vi "PXIe-SG.vi"() -> (0 "error out":errorcluster)   [LabVIEW 2022 SP3]
uses:
  Device ID port info.ctl
  Sub_vis/Upload Data.ctl
  <vilib>/DAQmx/read.llb/DAQmx Read (Analog 2D DBL NChan NSamp).vi
  Globals/Meas_global.vi
  <vilib>/DAQmx/miscellaneous.llb/DAQmx Fill In Error Info.vi
  <resource>/objmgr/daqmx.rc
panel:
  out "combinedTasks":string[](array[string])
  out "Device port info":T1[](array[typedef])
  out "FsReq":dbl=2000.0
  out "FsRead":dbl=2000.0000006348273 format="%#_11g"
  out "AuditTrail":string[](array[string])=["Clear Task", "Setup Channels etc", "Start Task", "Take data", "End"]
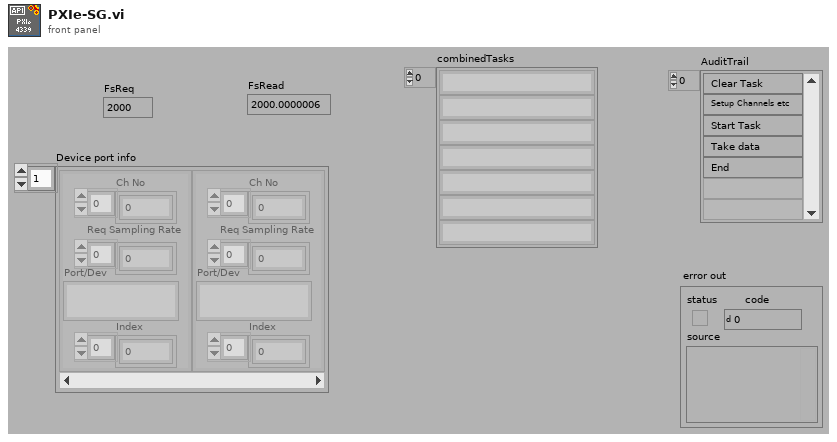
[diagram p1: front panel]
types:
  T1 = typedef "Device ID port info.ctl" = cluster{"Ch No":i16[], "Req Sampling Rate":dbl[], "Port":string, "Index":i32[]}
  T2 = typedef "Analysis_info_cluster.ctl" = cluster{"Colour":u32, "Inst type":T3, "Inst name":string, "Symbol":string, "Code name":string, "Extra Info":string, "Inst Array":T4, "U":dbl, "u^2":dbl, "u^3":dbl, "u^4":dbl, "Skew_u":dbl, "Kurt_u":dbl, "Sd Error in Mean":dbl, "% u'/U":dbl, "X":dbl, "Y":dbl, "Z":dbl, "Timescale integral Estimate":dbl, "Sd Error in Variance":dbl, "Calib File":path, "Calib Constants":dbl[], "Output Position":bool, "Stats":enum16{"None", "Basic", "Full"}, "Av Sampling Rate":dbl, "Av No of Samples":dbl, "Total Meas Time (s)":dbl, "OrigChName":string, "Max value":dbl, "Min value":dbl, "Req Sample Rate Hz":dbl, "Sync Delay Time (s)":dbl, "Ch No":i16, "Device":string, "Use Latest Calib":bool, "Port":string, "Metadata Ch Names":string[], "Metadata Ch Values":string[], "Label":string, "chState":T5, "Point Drift":dbl, "inputConfig":string}
  T3 = typedef "Inst_type.ctl" = enum16{"Raw voltage", "Raw with zero offsetting", "Propeller anemometer", "Pressure Transducer", "Pitot-static tube", "Hot wire", "Cross wire 1", "Cross wire 2", "Generic Linear", "Generic Polynomial", "Generic BackPoly", "Fast FID", "Thermocouple", "Cold wire", "Pulsed Wire", "LDA Vel", "LDA Tran time", "LDA Arr time", "Microphone"}
  T4 = typedef "Instrument_Array.ctl" = enum16{"PWA", "LDA", "Analogue"}
  T5 = typedef "channelState.ctl" = enum32{"No Selection", "Solo", "Mute"}
  T6 = typedef "Upload Data.ctl" = enum16{"Voltage Array", "Time Trace Cluster"}
  T7 = typedef "Rendezvous RefNum" = refnum<k1>
  T8 = typedef "Setup.ctl" = enum16{"Run Program", "Show Setup", "Save Current Setup", "Setup Front Panel"}
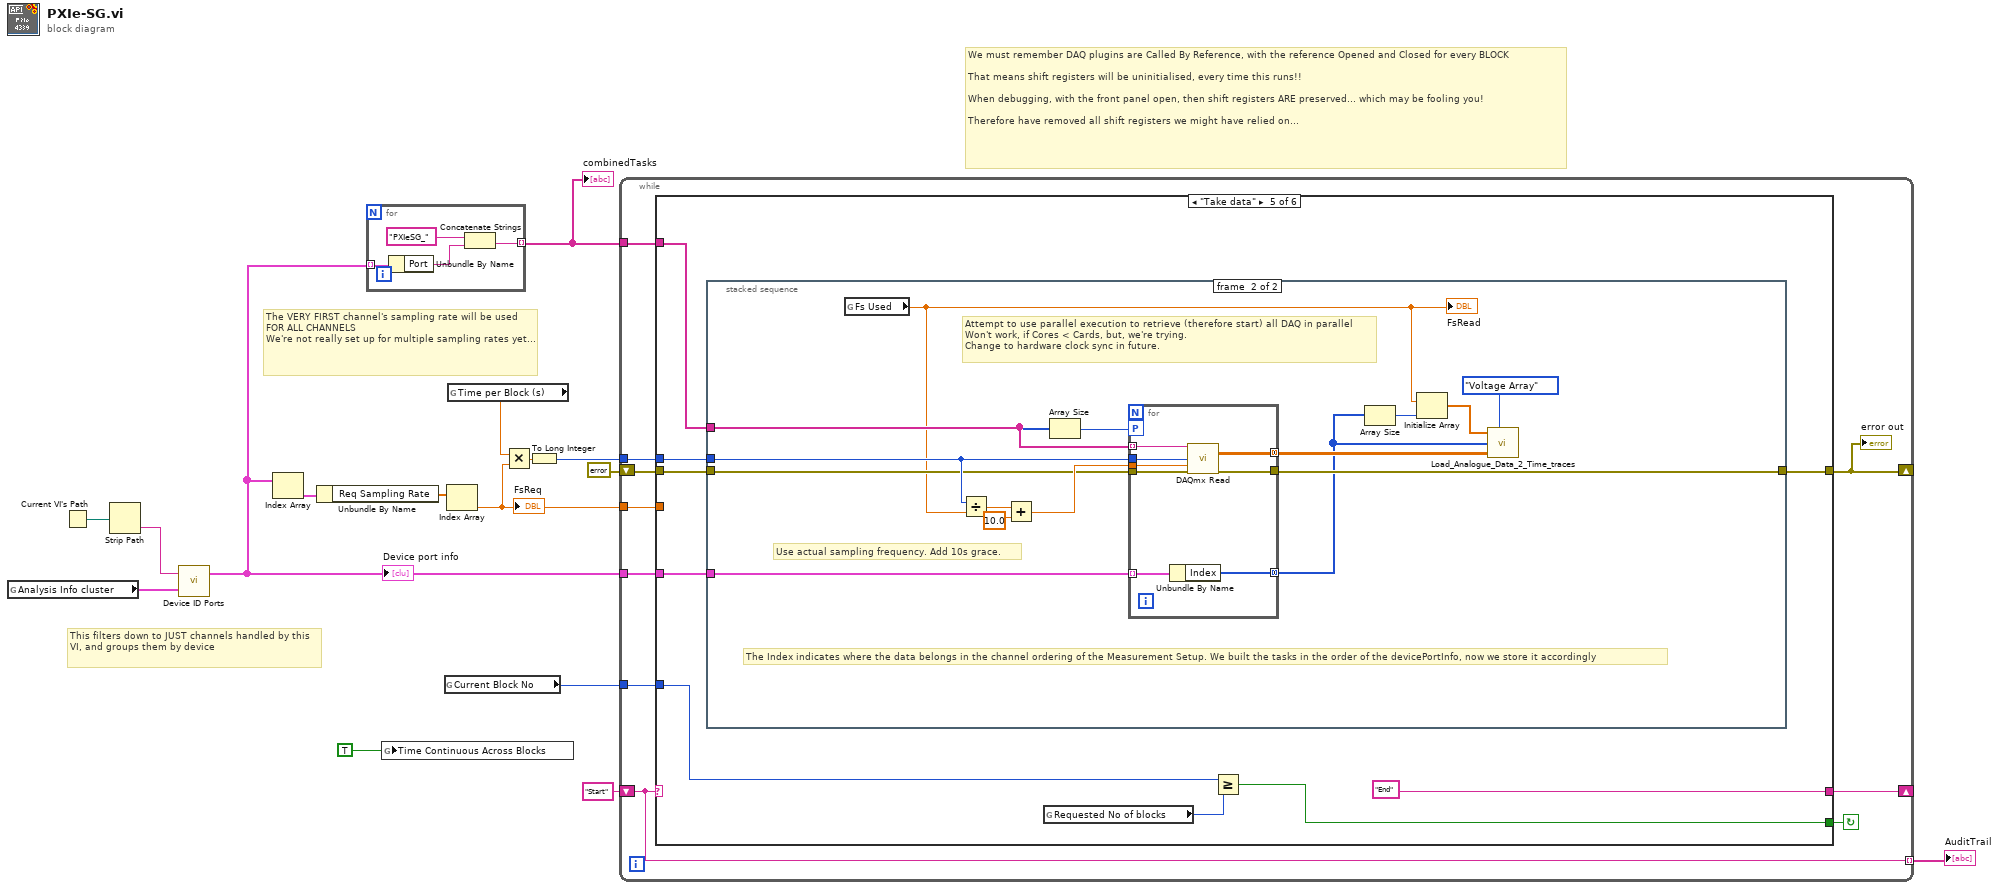
[diagram p0: block diagram]
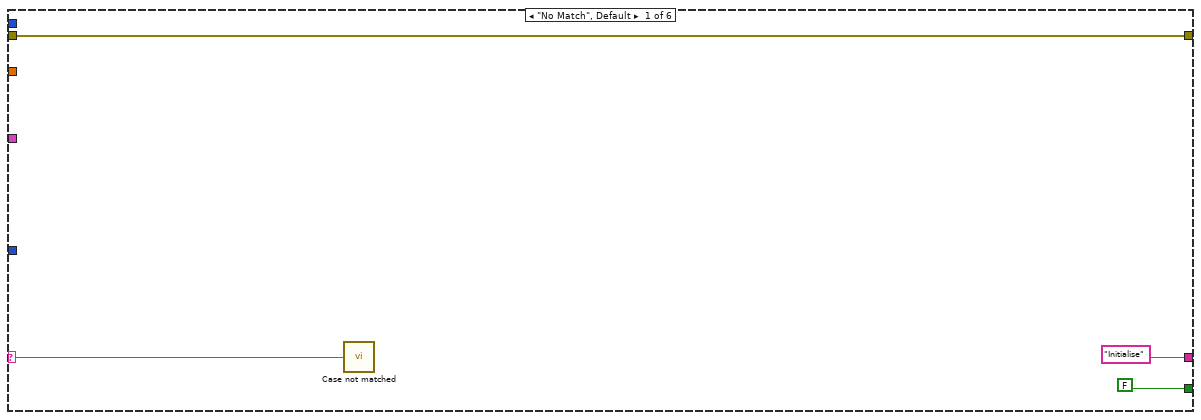
[diagram p2: hidden frame]
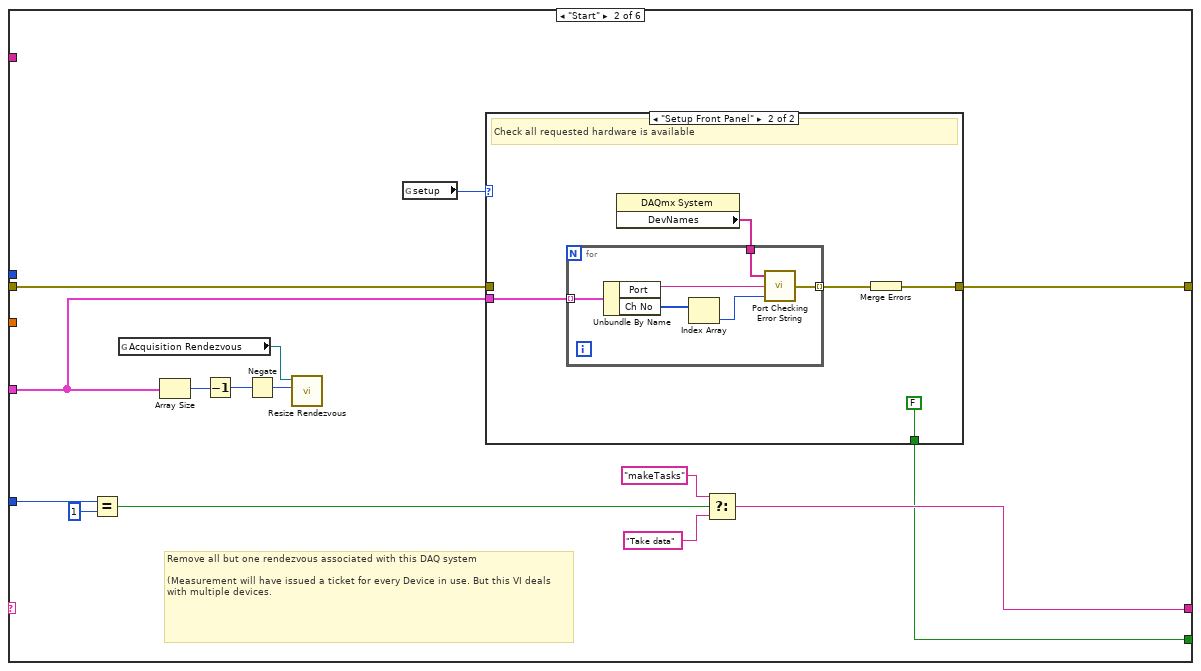
[diagram p3: hidden frame]
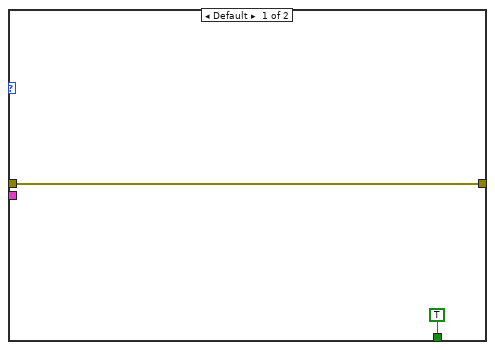
[diagram p4: hidden frame]
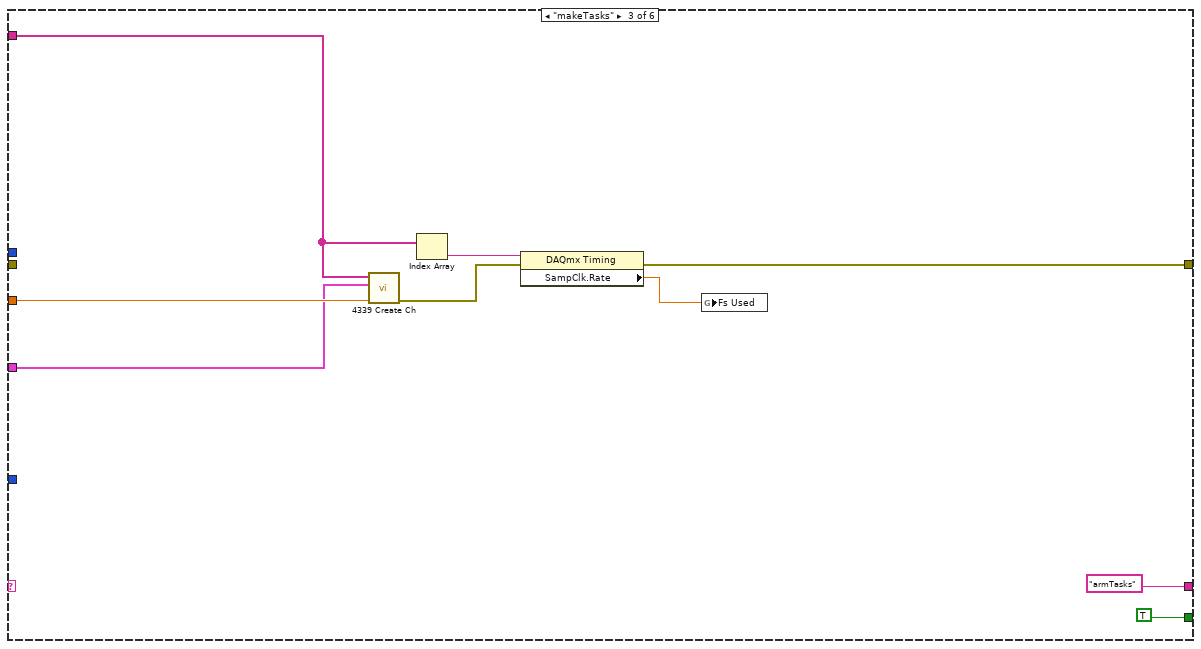
[diagram p5: hidden frame]
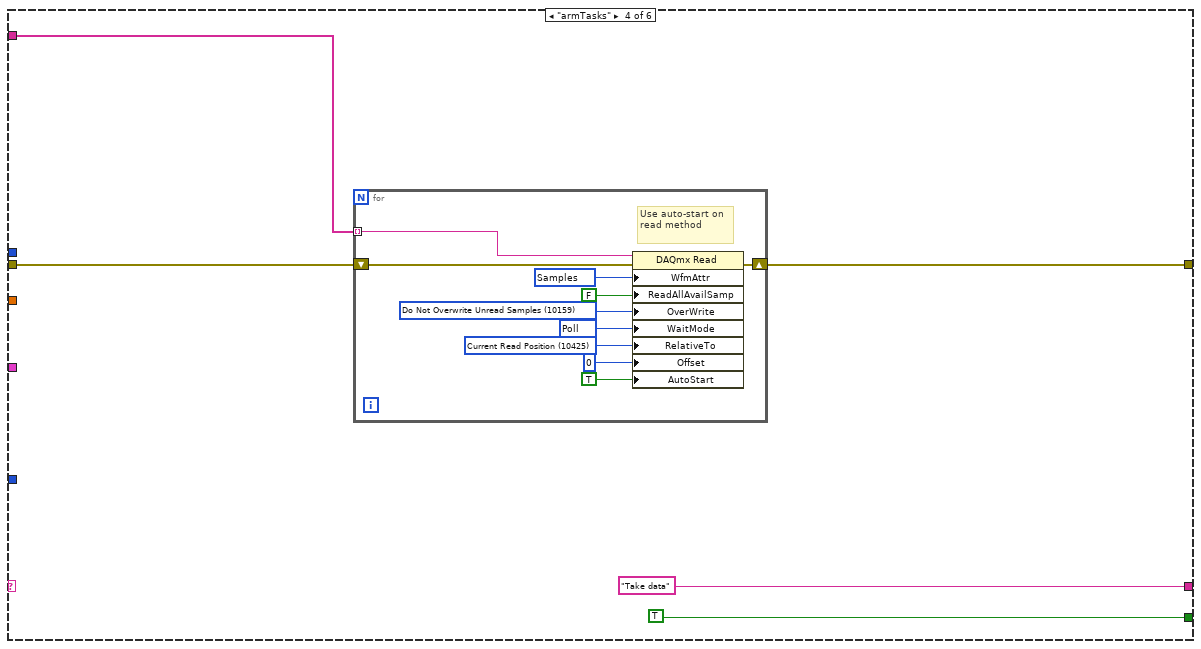
[diagram p6: hidden frame]
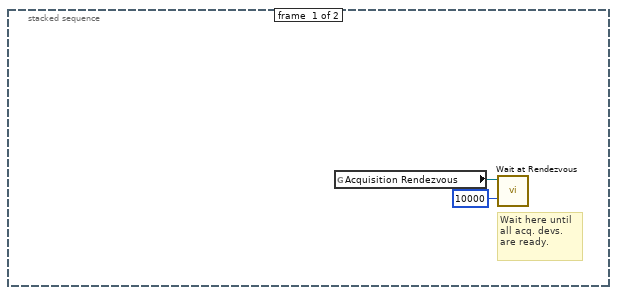
[diagram p7: hidden frame]
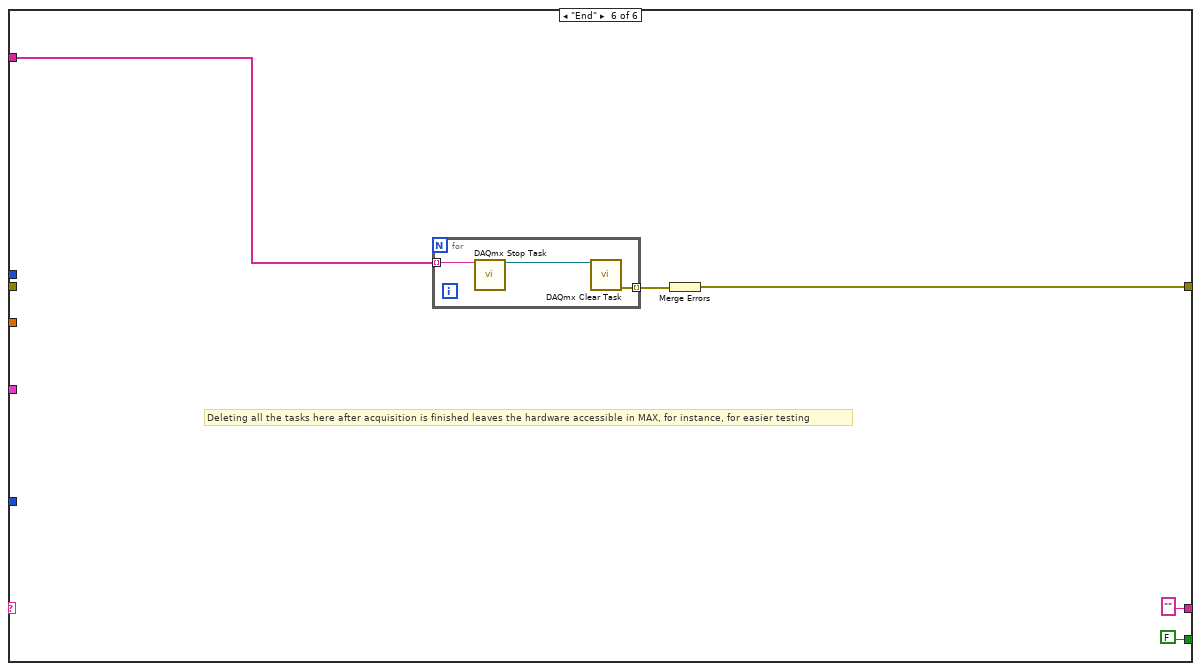
[diagram p8: hidden frame]
diagram:
  # "We must remember DAQ plugins are Called By Reference, with the reference Opened and Closed for every BLOCK\n\nThat means shift registers will be uninitialised, every time this runs!!\n\nWhen debugging, with the front panel open, then shift registers ARE preserved... which may be fooling you!\n\nTherefore have removed all shift registers we might have relied on..."
  # "The VERY FIRST channel's sampling rate will be used FOR ALL CHANNELS\nWe're not really set up for multiple sampling rates yet..."
  # "This filters down to JUST channels handled by this VI, and groups them by device"
  n1 = global read "Meas_global.vi" "Analysis Info cluster"() -> (w7:T2[])
  n2 = Current VI's Path() -> (path=w11:path)
  n3 = Strip Path(path=w11) -> (name=w10:string)  [unwired: 1 out]
  n4 = call "Device ID Ports.vi"("Analysis Info cluster"=w7, "DAQdeviceType"=w10) -> ("Device port info"=w2:T1[])  [unwired: 1 out]
  "Device port info" <- w2
  n5 = Index Array(array=w2) -> (element=w6:T1)  [unwired: 1 in]
  n6 = Unbundle By Name(w6) -> ("Req Sampling Rate"=w5:dbl[])
  n7 = for {
    tunnel: [w18] -> w1 mode=indexing
    tunnel: w2 -> [w17] mode=indexing
    n8 = Unbundle By Name(w17) -> ("Port"=w19:string)
    n9 = Concatenate Strings("PXIeSG_" ("new task name"), w19) -> (w18:string)
  }
  "combinedTasks" <- w1
  n10 = global write "Meas_global.vi" "Time Continuous Across Blocks"(TRUE ("Time Continuous across Blocks")) -> ()
  n11 = global read "Meas_global.vi" "Current Block No"() -> (w8:i32)
  n12 = Index Array(array=w5) -> (element=w4:dbl)  [unwired: 1 in]
  "FsReq" <- w4
  n13 = global read "Meas_global.vi" "Time per Block (s)"() -> (w9:dbl)
  n14 = Multiply(x=w9, y=w4) -> (x*y=w12:dbl)
  n15 = To Long Integer(number=w12) -> (32bit integer=w15:i32)
  n16 = while {
    shift-left: "Start" -> [w23]
    shift-right: [w27] -> _
    shift-right: [w22] -> _
    shift-left: errorcluster {"status"=FALSE, "code"=0, "source"=""} ("error out") -> [w30]
    tunnel: w15 -> [w29]
    tunnel: w8 -> [w28]
    tunnel: [w23] -> w14 mode=indexing
    tunnel: w2 -> [w25]
    tunnel: w4 -> [w24]
    tunnel: w1 -> [w21]
    stop <- w26 continue-if-true
    n17 = case shown="\"Take data\"" w23 {
      selector: w23 -> [w31 _ _ _ _ _]
      tunnel: [FALSE w44 TRUE TRUE w90 FALSE] -> w26
      tunnel: ["Initialise" w48 "armTasks" "Take data" "End" "" ("f")] -> w27
      tunnel: w30 -> [w32 w35 _ w72 w95 _]
      tunnel: w29 -> [_ _ _ _ w93 _]
      tunnel: w28 -> [_ w47 _ _ w87 _]
      tunnel: w21 -> [_ _ w65 w73 w91 w123]
      tunnel: w25 -> [_ w36 w66 _ w89 _]
      tunnel: w24 -> [_ _ w67 _ _ _]
      tunnel: [w32 w45 w68 w74 w92 w121] -> w22
      frame "No Match", Default {
        n18 = call "Case not matched.vi"("Case Name not Matched"=w31) -> ()
      }
      frame "Start" {
        # "Remove all but one rendezvous associated with this DAQ system\n\n(Measurement will have issued a ticket for every Device in use. But this VI deals with multiple devices."
        n19 = Equal?(x=w47, y=1) -> (x = y?=w41:bool)
        n20 = global read "Meas_global.vi" "Acquisition Rendezvous"() -> (w37:T7)
        n21 = Array Size(array=w36) -> (size(s)=w40:i32)
        n22 = Decrement(x=w40) -> (x-1=w39:i32)
        n23 = Negate(x=w39) -> (-x=w38:i32)
        n24 = call <vilib>:"Resize Rendezvous.vi"("size change (0)"=w38, "rendezvous"=w37) -> ()  [unwired: 3 in, 3 out]
        n25 = global read "Meas_global.vi" "setup"() -> (w46:T8)
        n26 = case shown="\"Setup Front Panel\"" w46 {
          tunnel: [w50 w52] -> w45
          tunnel: [TRUE FALSE] -> w44
          tunnel: w36 -> [_ w53]
          tunnel: w35 -> [w50 _]
          frame Default {
          }
          frame "Setup Front Panel" {
            # "Check all requested hardware is available"
            n27 = property class="DAQmx System"() -> ("DevNames"=w56:tag[])  [unwired: 2 in, 2 out]
            n28 = for {
              tunnel: w56 -> [w62]
              tunnel: [w61] -> w55 mode=indexing
              tunnel: w53 -> [w60] mode=indexing
              n29 = Unbundle By Name(w60) -> ("Port"=w59:string, "Ch No"=w58:i16[])
              n30 = Index Array(array=w58) -> (element=w57:i16)  [unwired: 1 in]
              n31 = call "Port Checking Error String.vi"("Ch Index"=w57, "Port"=w59, "Available Ports"=w62) -> ("error out"=w61:errorcluster)  [unwired: 1 in]
            }
            n32 = Merge Errors(w55) -> (w52:errorcluster)
          }
        }
        n33 = Select(t="makeTasks", s=w41, f="Take data") -> (s? t:f=w48:string)
      }
      frame "makeTasks" {
        n34 = call "4339 Create Ch.vi"("sampleRate"=w67, "Device port info"=w66, "taskNamesIn"=w65) -> ("error out"=w69:errorcluster)  [unwired: 8 in]
        n35 = Index Array(array=w65) -> (element=w64:string)  [unwired: 1 in]
        n36 = property class="DAQmx Timing"(reference=w64, error in=w69) -> (error out=w68:errorcluster, "SampClk.Rate"=w63:dbl)  [unwired: 1 out]
        n37 = global write "Meas_global.vi" "Fs Used"(w63) -> ()
      }
      frame "armTasks" {
        n38 = for {
          tunnel: w73 -> [w78] mode=indexing
          shift-right: [w79] -> w74
          shift-left: w72 -> [w77]
          w82 = 10425 items=["First Sample"=10424, "Current Read Position"=10425, "Reference Trigger"=10426, "First Pretrigger Sample"=10427, "Most Recent Sample"=10428] ("RelativeTo")
          w83 = 12524 items=["Wait For Interrupt"=12523, "Poll"=12524, "Yield"=12525, "Sleep"=12547] ("WaitMode")
          w84 = 10159 items=["Overwrite Unread Samples"=10252, "Do Not Overwrite Unread Samples"=10159] ("OverWrite")
          w86 = 10287 items=["Samples"=10287, "Samples and Timing"=10140, "Samples, Timing, and Attributes"=10141] ("WfmAttr")
          # "Use auto-start on read method"
          n39 = property class="DAQmx Read"(reference=w78, error in=w77, "WfmAttr"=w86, "ReadAllAvailSamp"=FALSE, "OverWrite"=w84, "WaitMode"=w83, "RelativeTo"=w82, "Offset"=0, "AutoStart"=TRUE) -> (error out=w79:errorcluster)  [unwired: 1 out]
        }
      }
      frame "Take data" {
        n40 = stacked-sequence {
          tunnel: w95 -> [_ w105]
          tunnel: w93 -> [_ w107]
          tunnel: [_ w104] -> w92
          tunnel: w91 -> [_ w102]
          tunnel: w89 -> [_ w101]
          frame #0 {
            # "Wait here until all acq. devs. are ready."
            n41 = global read "Meas_global.vi" "Acquisition Rendezvous"() -> (w97:T7)
            n42 = call <vilib>:"Wait at Rendezvous.vi"("ms timeout (-1)"=10000, "rendezvous"=w97) -> ()  [unwired: 3 in, 3 out]
          }
          frame #1 {
            # "Attempt to use parallel execution to retrieve (therefore start) all DAQ in parallel\nWon't work, if Cores < Cards, but, we're trying.\nChange to hardware clock sync in future."
            # "Use actual sampling frequency. Add 10s grace."
            # "The Index indicates where the data belongs in the channel ordering of the Measurement Setup. We built the tasks in the order of the devicePortInfo, now we store it accordingly"
            n43 = global read "Meas_global.vi" "Fs Used"() -> (w98:dbl)
            "FsRead" <- w98
            n44 = Divide(x=w107, y=w98) -> (x/y=w112:dbl)
            n45 = Add(x=w112, y=10.0) -> (x+y=w106:dbl)
            n46 = Array Size(array=w102) -> (size(s)=w103:i32)
            n47 = for {
              tunnel: w105 -> [w120]
              tunnel: w106 -> [w118]
              tunnel: w107 -> [w117]
              tunnel: [w119] -> w104
              tunnel: w102 -> [w116] mode=indexing
              workers-P: w103 -> [_]
              tunnel: [w115] -> w100 mode=concatenating
              tunnel: w101 -> [w114] mode=indexing
              tunnel: [w113] -> w99 mode=concatenating
              n48 = Unbundle By Name(w114) -> ("Index"=w113:i32[])
              n49 = call-poly <vilib>:"DAQmx Read.vi"("task/channels in"=w116, "number of samples per channel"=w117, "timeout"=w118, "error in"=w120) -> ("data"=w115:dbl[][], "error out"=w119:errorcluster)  [unwired: 10 out]
            }
            n50 = Array Size(array=w99) -> (size(s)=w110:i32)
            n51 = Initialize Array(w98, w110) -> (w109:dbl[])
            n52 = call "Load_Analogue_Data_2_Time_traces.vi"("Sampling Rate (Hz)"=w109, "Mode"=Upload_Data."Voltage Array", "Index"=w99, "Voltage Array"=w100) -> ()  [unwired: 3 in]
          }
        }
        n53 = global read "Meas_global.vi" "Requested No of blocks"() -> (w88:i32)
        n54 = Greater Or Equal?(x=w87, y=w88) -> (x >= y?=w90:bool)
      }
      frame "End" {
        # "Deleting all the tasks here after acquisition is finished leaves the hardware accessible in MAX, for instance, for easier testing"
        n55 = for {
          tunnel: w123 -> [w128] mode=indexing
          tunnel: [w126] -> w122 mode=indexing
          n56 = call <vilib>:"DAQmx Stop Task.vi"("task/channels in"=w128) -> ("task out"=w127:refnum<k21>)  [unwired: 13 in, 1 out]
          n57 = call <vilib>:"DAQmx Clear Task.vi"("task in"=w127) -> ("error out"=w126:errorcluster)  [unwired: 1 in, 13 out]
        }
        n58 = Merge Errors(w122) -> (w121:errorcluster)
      }
    }
    "error out" <- w22
  }
  "AuditTrail" <- w14
